vi "Create JSON Schema Header.vi"(8 "error in (no error)":errorcluster, 10 "Description":string, 11 "Title":string) -> (0 "error out":errorcluster, 3 "JSON Schema out":string)   [LabVIEW 2023, in "JSON Schema Generator.lvlib"]
uses:
  JSON Schema Generator.lvlib
  3ef15e4a-16dd-4668-bce3-ec6b426eb69a.vi
  407c657b-ac49-4f70-a0b2-c47d1b969b7f.vi
  <vilib>/JDP Science/JSONtext/Variant to JSON Text.vi
  <vilib>/JDP Science/JSONtext/LVClass Serializer/JSONtext LVClass Serializer.lvclass
  <vilib>/JDP Science/JSONtext/JSONtext.lvlib
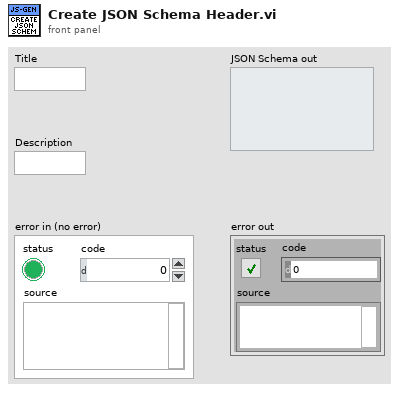
[diagram p1: front panel]
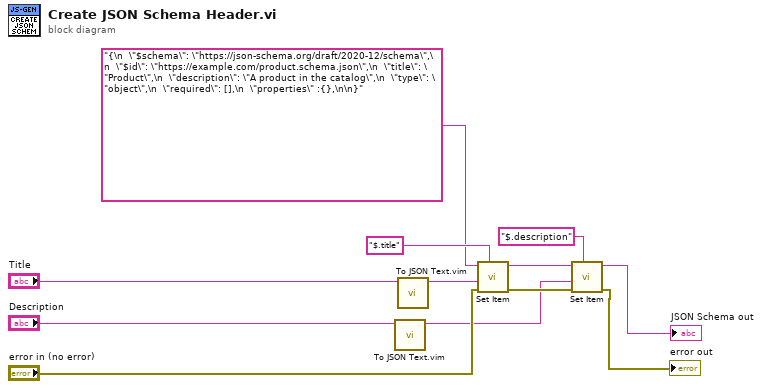
[diagram p0: block diagram]
diagram:
  n1 = call "To JSON Text.vim"("Anything"="Description") -> ("<JSON>"=w1:string)  [unwired: 9 in, 1 out]
  n2 = call "To JSON Text.vim"("Anything"="Title") -> ("<JSON>"=w10:string)  [unwired: 9 in, 1 out]
  n3 = call <vilib>:"Set Item.vi"("$Path or Item Name"="$.title", "error in (no error)"="error in (no error)", "JSON to Insert"=w10, "JSON"="{\n  \"$schema\": \"https://json-schema.org/draft/2020-12/schema\",\n  \"$id\": \"https://example.com/product.schema.json\",\n  \"title\": \"Product\",\n  \"description\": \"A product in the catalog\",\n  \"type\": \"object\",\n  \"required\": [],\n  \"properties\" :{},\n\n}") -> ("error out"=w7:errorcluster, "<JSON>"=w5:string)  [unwired: 4 in, 1 out]
  n4 = call <vilib>:"Set Item.vi"("$Path or Item Name"="$.description", "error in (no error)"=w7, "JSON to Insert"=w1, "JSON"=w5) -> ("error out"=→"error out":errorcluster, "<JSON>"=→"JSON Schema out":string)  [unwired: 4 in, 1 out]
